vi "HeadingTrue.vi"() -> ()   [LabVIEW 2012]
panel:
  out "Target X":i32
  out "Target Y":i32
  out "X Array":dbl[](array[numeric])
  out "Y Array":dbl[](array[numeric])
  out "Desired Heading":i32
  out "Current Y":i32
  out "Current X":i32
  out "Current Heading":i32
  in  "FULLSTOP":bool
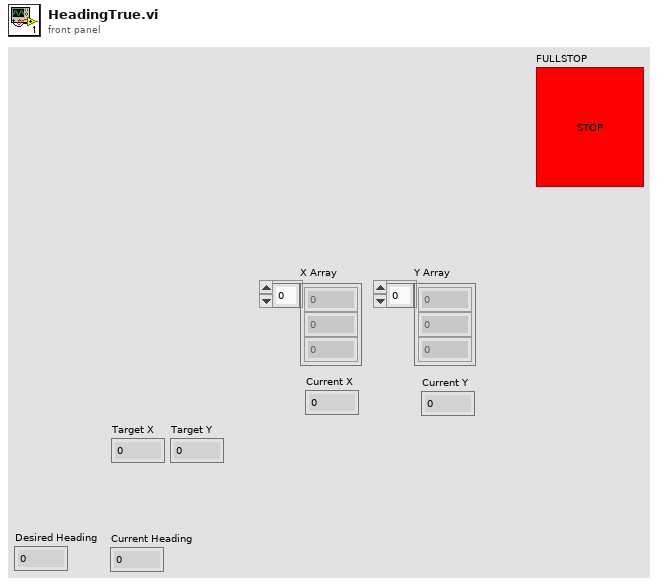
[diagram p1: front panel]
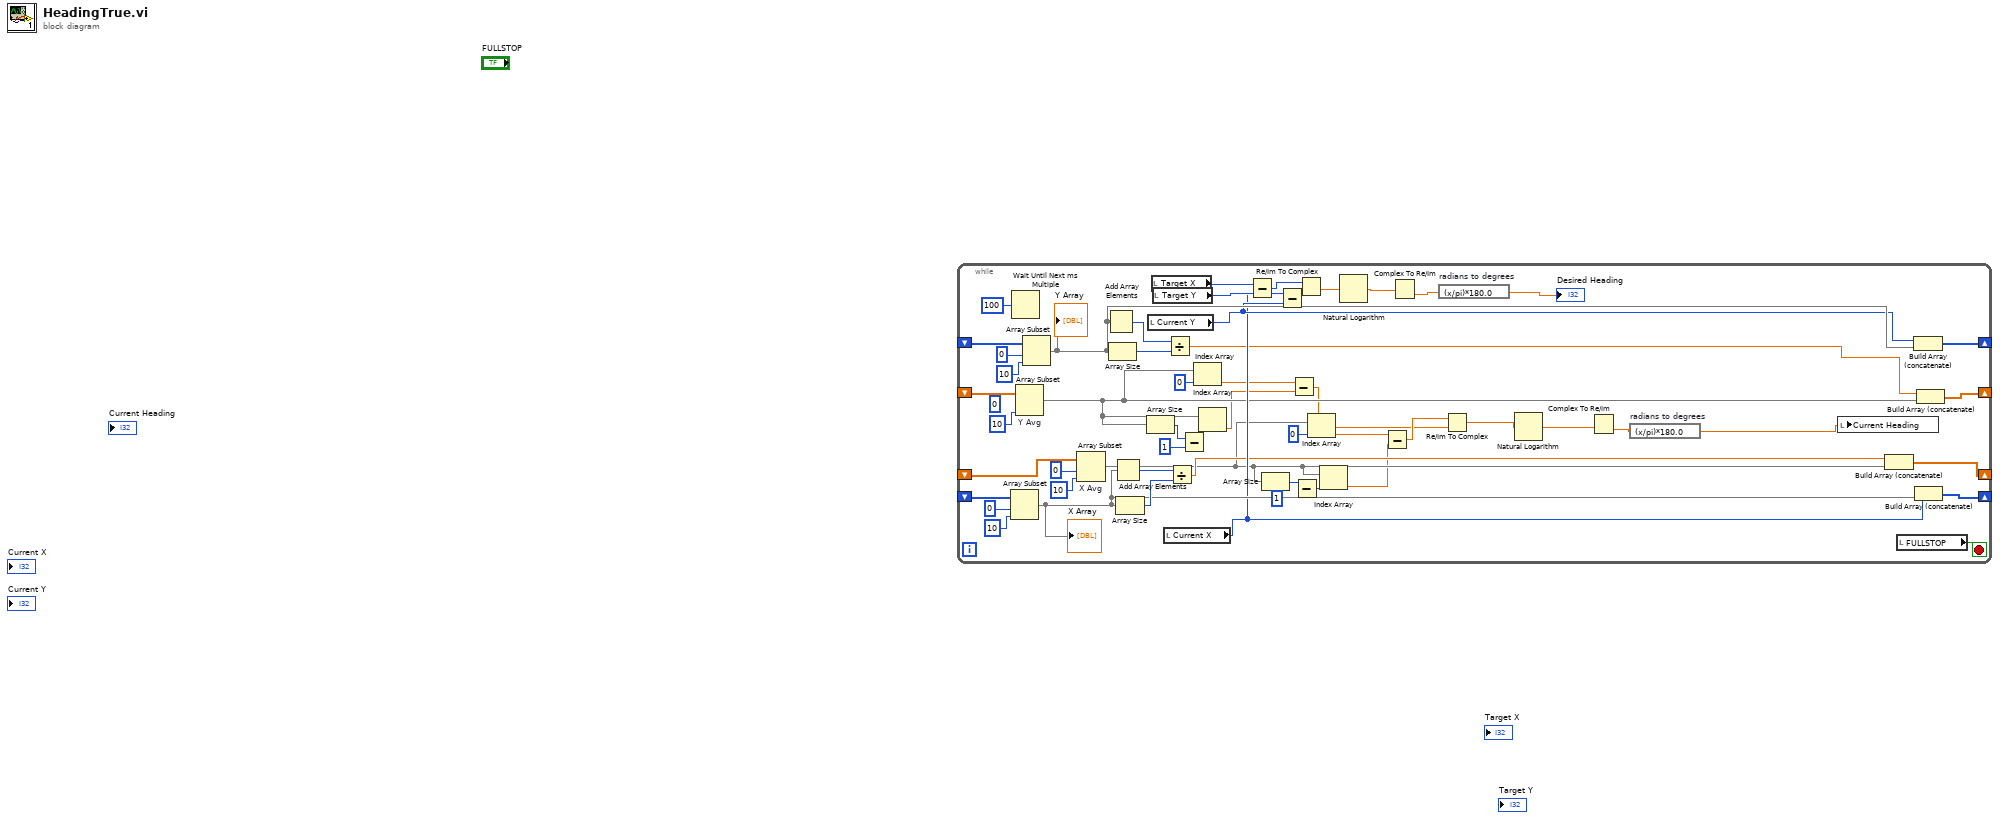
[diagram p0: block diagram]
diagram:
  n1 = while {
    shift-right: [w43] -> _
    shift-left: _ -> [w55]
    shift-right: [w42] -> _
    shift-left: _ -> [w50]
    shift-right: [w22] -> _
    shift-left: _ -> [w24]
    shift-right: [w29] -> _
    shift-left: _ -> [w26]
    stop <- w49 stop-if-true
    (unwired) 0 ("index")
    n2 = Array Subset(array=w55, index=0, length=10) -> (w41:i32[])
    "X Array" <- w41
    n3 = Wait Until Next ms Multiple(millisecond multiple=u32 100) -> ()  [unwired: 1 out]
    n4 = Array Subset "Y Avg"(array=w24, length=10) -> (w20:dbl[])  [unwired: 1 in]
    n5 = Array Subset(array=w50, index=0, length=10) -> (w40:i32[])
    "Y Array" <- w40
    n6 = Array Subset "X Avg"(array=w26, index=0, length=10) -> (w16:dbl[])
    n7 = Add Array Elements(numeric array=w40) -> (sum=w46:i32)
    n8 = Array Size(array=w40) -> (size(s)=w45:i32)
    n9 = Add Array Elements(numeric array=w41) -> (sum=w48:i32)
    n10 = Array Size(array=w41) -> (size(s)=w47:i32)
    n11 = Array Size(array=w20) -> (size(s)=w4:i32)
    n12 = local read "Current Y"() -> (w33:i32)
    n13 = local read "Target X"() -> (w32:i32)
    n14 = local read "Target Y"() -> (w44:i32)
    n15 = local read "Current X"() -> (w31:i32)
    n16 = Divide(x=w46, y=w45) -> (x/y=w23:dbl)
    n17 = Divide(x=w48, y=w47) -> (x/y=w30:dbl)
    n18 = Subtract(x=w4, y=1) -> (x-y=w3:i32)
    n19 = Index Array(array=w20, index=0) -> (element=w19:dbl)
    n20 = Index Array(array=w20, index=w3) -> (element=w18:dbl)
    n21 = Subtract(x=w32, y=w31) -> (x-y=w37:i32)
    n22 = Array Size(array=w16) -> (size(s)=w7:i32)
    n23 = Subtract(x=w44, y=w33) -> (x-y=w38:i32)
    n24 = Subtract(x=w19, y=w18) -> (x-y=w12:dbl)
    n25 = Subtract(x=w7, y=1) -> (x-y=w5:i32)
    n26 = Re/Im To Complex(1:w38, 2:w37) -> (0:w39:cdb)
    n27 = Index Array(array=w16, index=0) -> (element=w15:dbl)
    n28 = Index Array(array=w16, index=w5) -> (element=w14:dbl)
    n29 = Natural Logarithm(1:w39) -> (0:w36:cdb)
    n30 = Subtract(x=w15, y=w14) -> (x-y=w13:dbl)
    n31 = Complex To Re/Im(x + iy=w36) -> (y=w35:dbl)  [unwired: 1 out]
    n32 = expression code="(x/pi)*180.0" "radians to degrees"(w35) -> (→"Desired Heading":dbl)
    n33 = Re/Im To Complex(1:w12, 2:w13) -> (0:w11:cdb)
    n34 = Natural Logarithm(1:w11) -> (0:w10:cdb)
    n35 = Complex To Re/Im(x + iy=w10) -> (y=w9:dbl)  [unwired: 1 out]
    n36 = expression code="(x/pi)*180.0" "radians to degrees"(w9) -> (w8:dbl)
    n37 = local write "Current Heading"(w8) -> ()
    n38 = Build Array (concatenate)(w30, w16) -> (w29:dbl[])
    n39 = local read "FULLSTOP"() -> (w49:bool)
    n40 = Build Array (concatenate)(w33, w40) -> (w42:i32[])
    n41 = Build Array (concatenate)(w31, w41) -> (w43:i32[])
    n42 = Build Array (concatenate)(w23, w20) -> (w22:dbl[])
  }
